vi "ad ioctl.vi"(7 "size":i32, 8 "error in (no error)":errorcluster, 9 "p":u32, 10 "ioc":i32, 11 "adh":i32) -> (0 "error out":errorcluster, 1 "p out":u32, 3 "function return":i32)   [LabVIEW 2021, in "libad4.lvlib"]
doc: "LIBAD4 function: ad_ioctl (int32_t adh, int32_t ioc, void *p, int32_t size);\n\nUndocumented function."
uses:
  <userlib>/libad4/libad4.lvlib
  <userlib>/libad4/libad4.dll
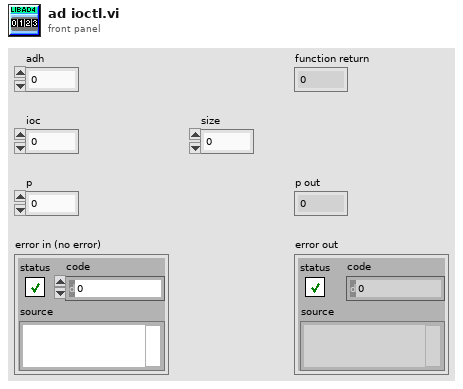
[diagram p1: front panel]
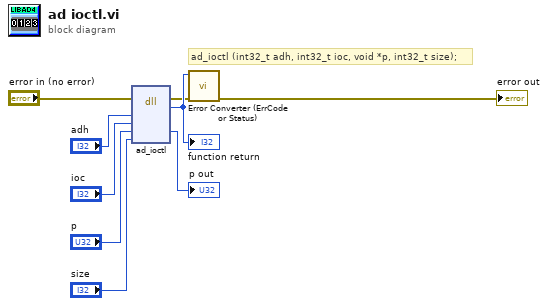
[diagram p0: block diagram]
diagram:
  # "ad_ioctl (int32_t adh, int32_t ioc, void *p, int32_t size);"
  n1 = dll-call lib="C:/Program Files/National Instruments/LabVIEW 2021/user.lib/libad4/libad4.*" fn="ad_ioctl"(error in="error in (no error)", "adh"="adh", "ioc"="ioc", "p"="p", "size"="size") -> (error out=w2:errorcluster, w9:i32, "p"=→"p out":u32)  [unwired: 5 in, 1 out]
  "function return" <- w9
  n2 = call <userlib>:"Error Converter (ErrCode or Status).vi"("error in (no error)"=w2, "error code"=w9) -> ("error out"=→"error out":errorcluster)  [unwired: 9 in]
